vi "SetBottomPaneSize.vi"(8 "error in (no error)":errorcluster, 9 "Bottom Pane Size":i32, 10 "Front Panel":refnum<vi>, 11 "Splitters":T1) -> (0 "error out":errorcluster)   [LabVIEW 2022 SP3, in "PentaPanesLibrary.lvlib" / "PentaPanes.lvclass"]
uses:
  PentaPanes.lvclass
  SplittersCluster.ctl
panel:
  out "In Range?":bool
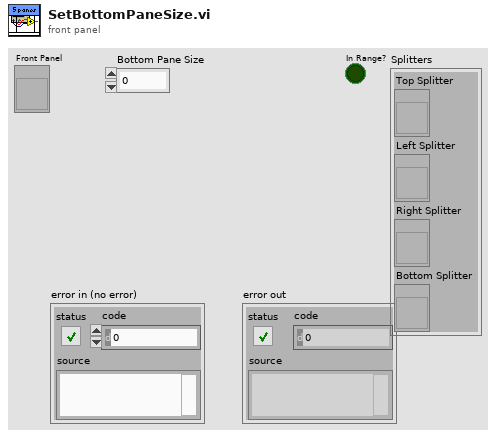
[diagram p1: front panel]
types:
  T1 = typedef "PentaPanesLibrary.lvlib/PentaPanes.lvclass/SplittersCluster.ctl" = cluster{"Top Splitter":refnum<vi>, "Left Splitter":refnum<vi>, "Right Splitter":refnum<vi>, "Bottom Splitter":refnum<vi>}
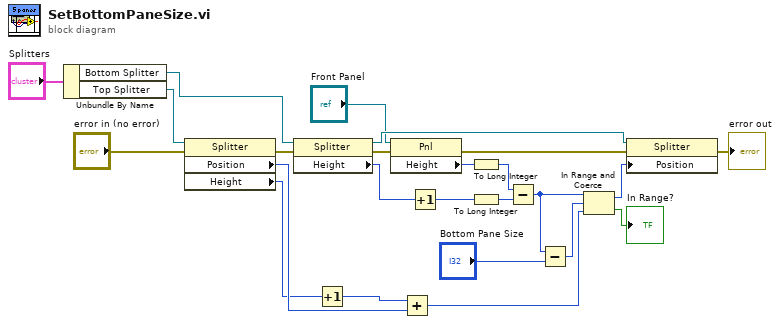
[diagram p0: block diagram]
diagram:
  n1 = Unbundle By Name("Splitters") -> ("Bottom Splitter"=w23:refnum<vi>, "Top Splitter"=w17:refnum<vi>)
  n2 = property class="Splitter"(reference=w17, error in="error in (no error)") -> (error out=w3:errorcluster, "Position"=w19:i32, "Height"=w6:u32)  [unwired: 1 out]
  n3 = property class="Splitter"(reference=w23, error in=w3) -> (reference out=w21:refnum<vi>, error out=w2:errorcluster, "Height"=w22:u32)
  n4 = Increment(x=w6) -> (x+1=w5:u32)
  n5 = property class="Pnl"(reference="Front Panel", error in=w2) -> (error out=w1:errorcluster, "Height"=w10:u32)  [unwired: 1 out]
  n6 = Add(x=w5, y=w19) -> (x+y=w18:u32)
  n7 = Increment(x=w22) -> (x+1=w12:u32)
  n8 = To Long Integer(number=w10) -> (32bit integer=w9:i32)
  n9 = To Long Integer(number=w12) -> (32bit integer=w11:i32)
  n10 = Subtract(x=w9, y=w11) -> (x-y=w16:i32)
  n11 = Subtract(x=w16, y="Bottom Pane Size") -> (x-y=w15:i32)
  n12 = In Range and Coerce(upper limit=w16, x=w15, lower limit=w18) -> (coerced(x)=w14:u32, In Range?=→"In Range?":bool)
  n13 = property class="Splitter"(reference=w21, error in=w1, "Position"=w14) -> (error out=→"error out":errorcluster)  [unwired: 1 out]
